vi "Coerce Engine Speed.vi"(0 "RPM Selection In":u16, 1 "RPM Array":dbl[](array[numeric]), 2 "Manual Desired RPM":dbl, 6 "Min Engine Speed in":dbl) -> (15 "Min Engine Speed out":dbl)   [LabVIEW 2013]
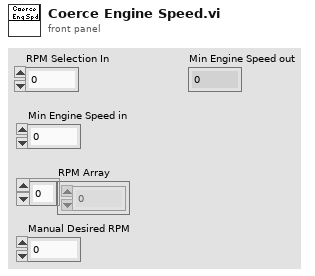
[diagram p1: front panel]
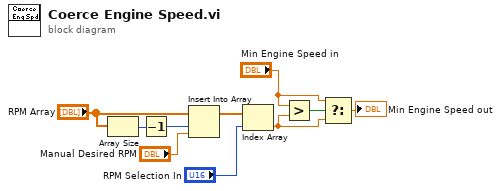
[diagram p0: block diagram]
diagram:
  n1 = Array Size(array="RPM Array") -> (size(s)=w2:i32)
  n2 = Decrement(x=w2) -> (x-1=w1:i32)
  n3 = Insert Into Array(array="RPM Array", index=w1, new element="Manual Desired RPM") -> (w5:dbl[])
  n4 = Index Array(array=w5, index="RPM Selection In") -> (element=w10:dbl)
  n5 = Greater?(x="Min Engine Speed in", y=w10) -> (0:w7:bool)
  n6 = Select(t="Min Engine Speed in", s=w7, f=w10) -> (s? t:f=→"Min Engine Speed out":dbl)
